vi "Reference.vi"(0 "file path (IN)":path, 1 "Project #":string, 2 "Request #":string, 3 "TEST #":string, 5 "error in (no error)":errorcluster, 6 "ICE":dbl) -> (7 "Ta (ns)":dbl, 9 "Tb (ns)":dbl, 11 "Irrm(A)":dbl, 13 "Erec (uj)":dbl, 14 "file path (OUT)":path, 15 "TRR (ns)":dbl, 16 "QRR (nc)":dbl, 17 "DONE":bool, 19 "error out":errorcluster)   [LabVIEW 2020]
uses:
  <vilib>/Analysis/NI_AALBase.lvlib
  <vilib>/measure/NI_MAPro.lvlib
  <vilib>/measure/mamon.llb/Trigger Detection for 1 Channel.vi
  <vilib>/Analysis/NI_AALPro.lvlib
  <vilib>/Analysis/1siggen.llb/Ramp Pattern by Samples.vi
panel:
  out "Erec: X-axis":dbl[](array[numeric])
  out "Erec: Y-axis":dbl[](array[numeric])
  out "Erec  : XY Graph":cluster{"X":dbl, "Y":dbl}[](graph)
  out "QRR Part2(RAMP): X-axis":dbl[](array[numeric])
  out "QRR Part2(RAMP): Y-axis":dbl[](array[numeric])
  out "QRR Part2(RAMP) : XY Graph":cluster{"X":dbl, "Y":dbl}[](graph)
  out "x-intercept of RAMP":dbl
  out "y-intercept":dbl
  out "slope":dbl
  out "QRR Part1(ICE): X-axis":dbl[](array[numeric])
  out "QRR Part1(ICE) : XY Graph":cluster{"X":dbl, "Y":dbl}[](graph)
  out "QRR Part1(ICE): Y-axis":dbl[](array[numeric])
  in  "Decision ?":bool
  out "25% Irrm Rise Edge":dbl
  out "0% Ice-Fall Edge":dbl
  out "Cursor a : Channel 1":dbl
  out "Cursor b : Channel 1":dbl
  out "Waveform Graph":waveform(dbl)[](graph)
  out "ON Region":waveform(dbl)[](graph) caption="Erec(uj)"
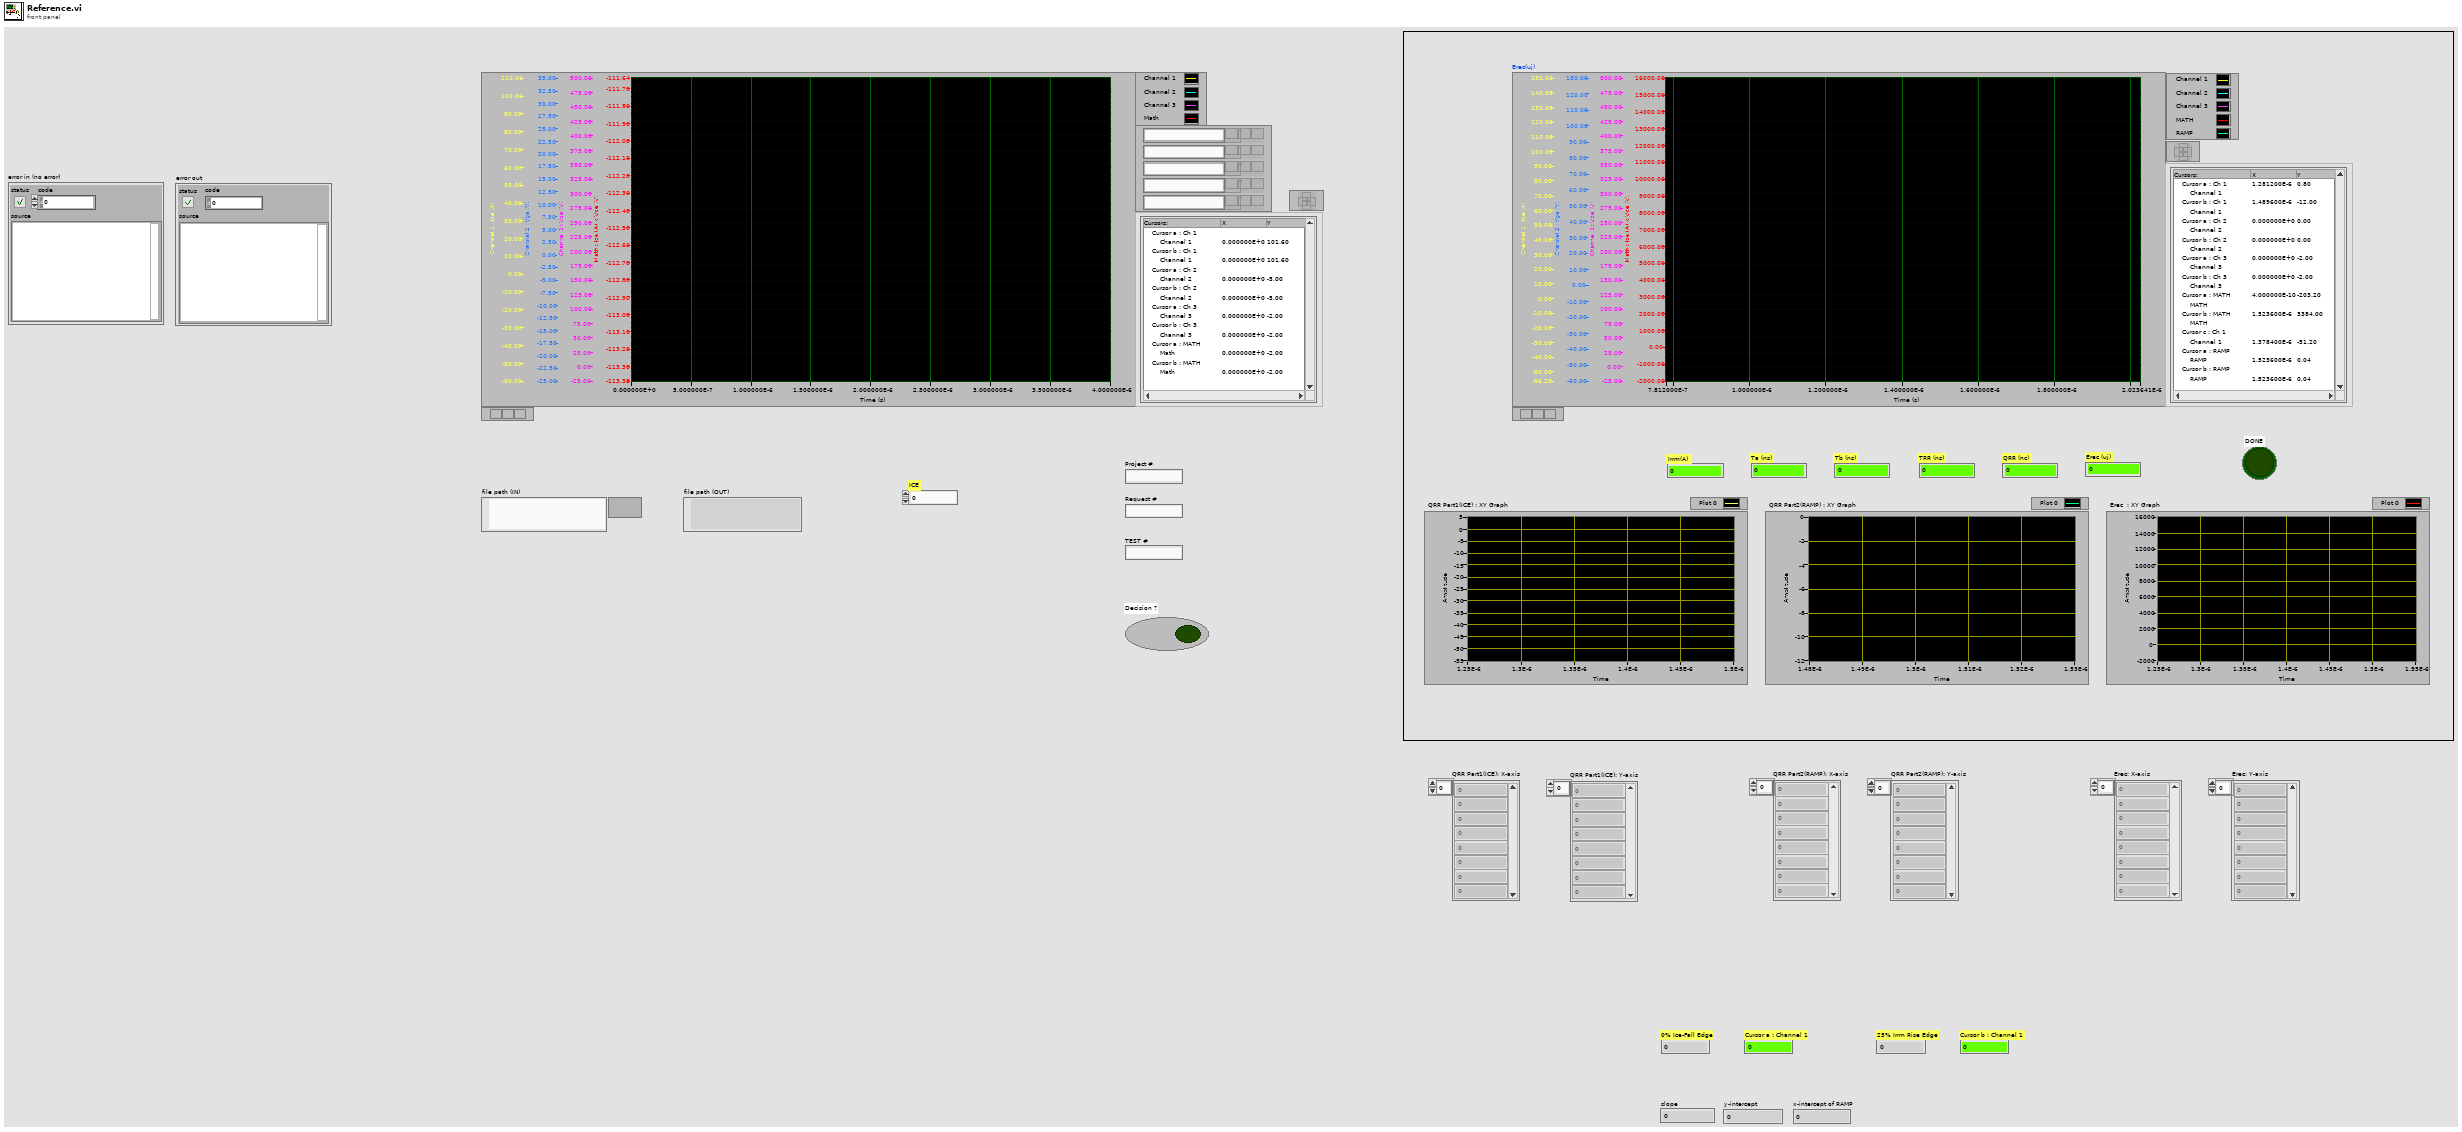
[diagram p1: front panel]
types:
  T1 = enum32{"Invalid", "Standard", "Closed", "Hidden", "Minimized", "Maximized"}
  T2 = typedef "imagedata.ctl" = cluster{"image type":i32, "image depth":i32, "image":u8[], "mask":u8[], "colors":u32[], "Rectangle":cluster{"left":i16, "top":i16, "right":i16, "bottom":i16}}
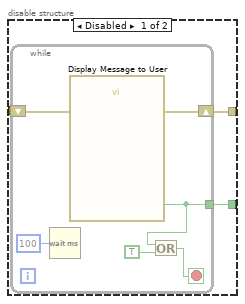
[diagram p3: hidden frame]
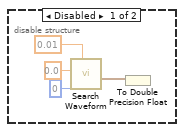
[diagram p7: hidden frame]
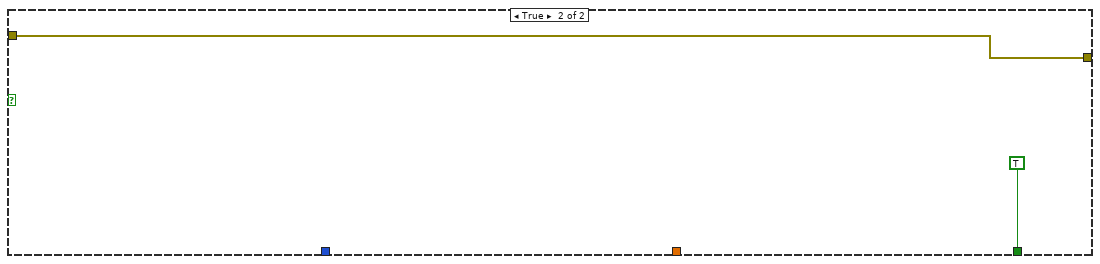
[diagram p9: hidden frame]
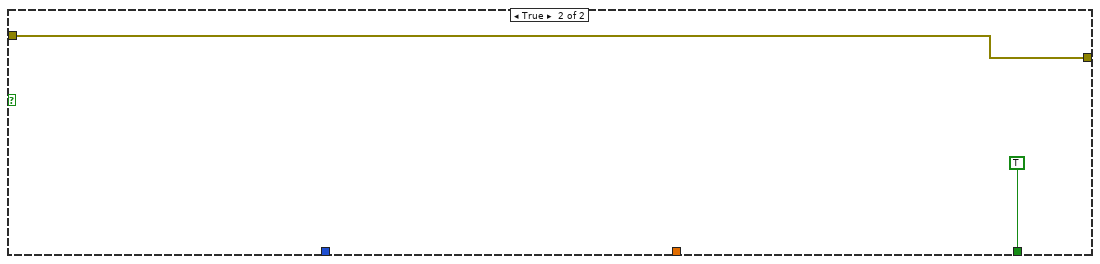
[diagram p10: hidden frame]
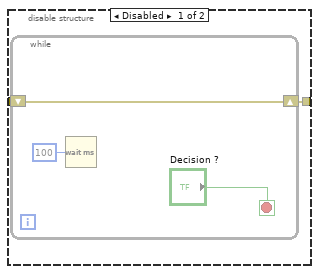
[diagram p12: hidden frame]
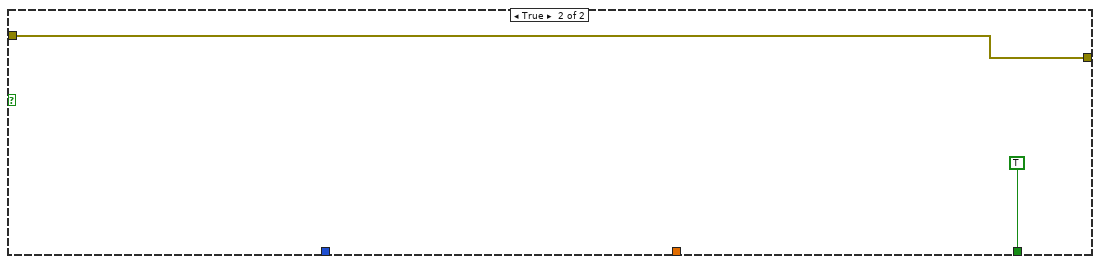
[diagram p13: hidden frame]
diagram:
  w31 = FALSE ("DONE Tdon")
  w16 = 0.0 ("Cursor a : Channel 1")
  w32 = errorcluster {"status"=FALSE, "code"=0, "source"=""} ("error out")
  w33 = waveform(dbl)[] [] ("Waveform Graph")
  n1 = local write "Cursor a : Channel 1"(w16) -> ()
  n2 = local write "Cursor b : Channel 1"(w16) -> ()
  n3 = local write "Decision ?"(w31) -> ()
  n4 = local write "error out"(w32) -> ()
  n5 = local write "error in (no error)"(w32) -> ()
  n6 = local write "DONE"(w31) -> ()
  n7 = local write "TRR (ns)"(w16) -> ()
  n8 = local write "QRR (nc)"(w16) -> ()
  n9 = local write "Waveform Graph"(w33) -> ()
  n10 = local write "ON Region"(w33) -> ()
  n11 = local write "Tb (ns)"(w16) -> ()
  n12 = local write "Erec (uj)"(w16) -> ()
  n13 = local write "Ta (ns)"(w16) -> ()
  n14 = local write "Irrm(A)"(w16) -> ()
  n15 = flat-sequence {
    tunnel: ["file path (IN)"] -> w37
    tunnel: [w38] -> w36
    tunnel: [w53] -> w35
    tunnel: [w52] -> w34
    tunnel: w37 -> [w55]
    tunnel: w36 -> [w54]
    tunnel: [w49] -> w20
    tunnel: [w48] -> w15
    tunnel: [w47] -> w14
    tunnel: [w46] -> w13
    tunnel: [w610] -> w12
    tunnel: w35 -> [w609]
    tunnel: w34 -> [w608]
    tunnel: [w608] -> w11
    tunnel: w20 -> [w607]
    tunnel: [w607] -> w9
    tunnel: w15 -> [w606]
    tunnel: [w606] -> w7
    tunnel: [w605] -> w5
    tunnel: w14 -> [w605]
    tunnel: [w604] -> w3
    tunnel: w13 -> [w604]
    tunnel: w12 -> [w624]
    tunnel: w11 -> [w634]
    tunnel: [w634] -> w10
    tunnel: w9 -> [w633]
    tunnel: [w633] -> w8
    tunnel: w7 -> [w632]
    tunnel: [w632] -> w6
    tunnel: w5 -> [w631]
    tunnel: [w631] -> w4
    tunnel: w3 -> [w630]
    tunnel: [w630] -> w2
    tunnel: [w623] -> w1
    tunnel: [w635] -> w24
    tunnel: w10 -> [w649]
    tunnel: [w649] -> w22
    tunnel: w8 -> [w640]
    tunnel: w6 -> [w636]
    tunnel: w4 -> [w637]
    tunnel: w2 -> [w639]
    tunnel: w1 -> [w641]
    tunnel: w24 -> [w764]
    tunnel: [w762] -> w23
    tunnel: w22 -> [w777]
    tunnel: [w777] -> w21
    tunnel: w23 -> [w779]
    tunnel: w21 -> [w778]
    frame #0 {
      n16 = control-ref of="This VI"() -> (w43:refnum<vi>)
      n17 = invoke class="VI" method="FP.Open"(reference=w43, error in="error in (no error)", "Activate"=TRUE ("Activate?"), "State"=T1."Maximized") -> (error out=w44:errorcluster)  [unwired: 1 in, 4 out]
      n18 = property class="VI"(reference=w43, error in=w44, "Front Panel.Closeable"=TRUE ("Front Panel Window:Closeable")) -> (error out=w38:errorcluster)  [unwired: 1 out]
    }
    frame #1 {
      n19 = while {
        tunnel: w55 -> [w128]
        shift-right: [w123] -> w53
        shift-left: w54 -> [w127]
        tunnel: [w125] -> w52
        tunnel: [w74] -> w51
        tunnel: [w73] -> w50
        tunnel: [w71] -> w48
        tunnel: [w70] -> w47
        tunnel: [w68] -> w46
        stop <- w122 stop-if-true
        n20 = flat-sequence {
          tunnel: [w158] -> w136
          tunnel: [w159] -> w135
          tunnel: w128 -> [w159]
          tunnel: w127 -> [w158]
          tunnel: w136 -> [w245]
          tunnel: w135 -> [w242]
          tunnel: [w193] -> w134
          tunnel: [w182] -> w121
          tunnel: [w179] -> w116
          tunnel: [w162] -> w93
          tunnel: [w161] -> w74
          tunnel: [w160] -> w73
          tunnel: w134 -> [w305]
          tunnel: [w305] -> w119
          tunnel: [w290] -> w118
          tunnel: w121 -> [w274]
          tunnel: [w268] -> w117
          tunnel: w116 -> [w270]
          tunnel: [w270] -> w115
          tunnel: [w269] -> w107
          tunnel: [w268] -> w106
          tunnel: [w264] -> w105
          tunnel: [w266] -> w104
          tunnel: [w267] -> w103
          tunnel: [w266] -> w96
          tunnel: w93 -> [w265]
          tunnel: [w264] -> w80
          tunnel: w119 -> [w361]
          tunnel: [w361] -> w102
          tunnel: w118 -> [w360]
          tunnel: [w360] -> w101
          tunnel: w117 -> [w359]
          tunnel: [w359] -> w100
          tunnel: [w331] -> w99
          tunnel: w115 -> [w331]
          tunnel: [w330] -> w98
          tunnel: w107 -> [w357]
          tunnel: [w357] -> w97
          tunnel: w106 -> [w339]
          tunnel: w105 -> [w338]
          tunnel: w104 -> [w337]
          tunnel: w103 -> [w336]
          tunnel: w96 -> [w329]
          tunnel: [w329] -> w95
          tunnel: w80 -> [w328]
          tunnel: [w328] -> w78
          tunnel: w102 -> [w374]
          tunnel: [w374] -> w113
          tunnel: w101 -> [w373]
          tunnel: [w373] -> w112
          tunnel: [w365] -> w111
          tunnel: w100 -> [w372]
          tunnel: [w372] -> w110
          tunnel: w99 -> [w371]
          tunnel: [w371] -> w109
          tunnel: w98 -> [w364]
          tunnel: [w364] -> w108
          tunnel: w97 -> [w369]
          tunnel: w95 -> [w363]
          tunnel: [w363] -> w94
          tunnel: [w362] -> w79
          tunnel: w78 -> [w362]
          tunnel: w113 -> [w389]
          tunnel: [w389] -> w92
          tunnel: w112 -> [w380]
          tunnel: [w380] -> w90
          tunnel: w111 -> [w387]
          tunnel: [w385] -> w88
          tunnel: w110 -> [w388]
          tunnel: [w388] -> w86
          tunnel: w109 -> [w375]
          tunnel: [w379] -> w84
          tunnel: w108 -> [w379]
          tunnel: w94 -> [w378]
          tunnel: [w378] -> w82
          tunnel: w79 -> [w377]
          tunnel: [w377] -> w77
          tunnel: [w376] -> w76
          tunnel: [w375] -> w75
          tunnel: w92 -> [w476]
          tunnel: [w476] -> w91
          tunnel: w90 -> [w475]
          tunnel: [w475] -> w89
          tunnel: w88 -> [w466]
          tunnel: [w465] -> w87
          tunnel: w86 -> [w474]
          tunnel: [w474] -> w85
          tunnel: w84 -> [w473]
          tunnel: [w473] -> w83
          tunnel: w82 -> [w472]
          tunnel: [w472] -> w81
          tunnel: w77 -> [w463]
          tunnel: w76 -> [w460]
          tunnel: w75 -> [w459]
          tunnel: [w459] -> w68
          tunnel: [w555] -> w133
          tunnel: w91 -> [w558]
          tunnel: [w558] -> w132
          tunnel: w89 -> [w557]
          tunnel: [w557] -> w131
          tunnel: w87 -> [w556]
          tunnel: w85 -> [w552]
          tunnel: [w552] -> w120
          tunnel: [w553] -> w114
          tunnel: w83 -> [w553]
          tunnel: w81 -> [w551]
          tunnel: w133 -> [w585]
          tunnel: w132 -> [w588]
          tunnel: [w588] -> w130
          tunnel: w131 -> [w575]
          tunnel: [w585] -> w129
          tunnel: w120 -> [w577]
          tunnel: w114 -> [w574]
          tunnel: [w575] -> w72
          tunnel: [w574] -> w69
          tunnel: w130 -> [w595]
          tunnel: w129 -> [w597]
          tunnel: [w596] -> w124
          tunnel: [w595] -> w125
          tunnel: w72 -> [w594]
          tunnel: [w594] -> w71
          tunnel: [w593] -> w70
          tunnel: w69 -> [w593]
          frame #0 {
            w155 = waveform(dbl)[] [] ("Waveform Graph")
            w151 = 0.0 ("Cursor a : Channel 1")
            w157 = FALSE ("DONE Tdon")
            n21 = local write "Cursor a : Channel 1"(w151) -> ()
            n22 = local write "TRR (ns)"(w151) -> ()
            n23 = local write "Cursor b : Channel 1"(w151) -> ()
            n24 = local write "Decision ?"(w157) -> ()
            n25 = local write "QRR (nc)"(w151) -> ()
            n26 = local write "Tb (ns)"(w151) -> ()
            n27 = local write "Irrm(A)"(w151) -> ()
            n28 = local write "Ta (ns)"(w151) -> ()
            n29 = local write "DONE"(w157) -> ()
            n30 = local write "QRR Part2(RAMP) : XY Graph"(cluster{"X":dbl, "Y":dbl}[] [] ("QRR : XY Graph")) -> ()
            n31 = local write "QRR Part2(RAMP): X-axis"(dbl[] [] ("QRR Area Y-axis")) -> ()
            n32 = local write "QRR Part2(RAMP): Y-axis"(dbl[] [] ("QRR Area X-axis")) -> ()
            n33 = local write "QRR Part1(ICE) : XY Graph"(cluster{"X":dbl, "Y":dbl}[] [] ("QRR : XY Graph")) -> ()
            n34 = local write "QRR Part1(ICE): Y-axis"(dbl[] [] ("QRR Area Y-axis")) -> ()
            n35 = local write "QRR Part1(ICE): X-axis"(dbl[] [] ("QRR Area X-axis")) -> ()
            n36 = Wait (ms)(milliseconds to wait=u32 200) -> ()  [unwired: 1 out]
            n37 = local write "Waveform Graph"(w155) -> ()
            n38 = local write "ON Region"(w155) -> ()
          }
          frame #1 {
            w183 = 0.0 ("number")
            w168 = waveform(dbl) {"t0"=timestamp(0 s since 1904-01-01), "dt"=1.0, "Y"=[]} ("element")
            # "t0"
            # "Channel 1"
            # "Channel 3"
            # "dt"
            # "Ch1"
            n39 = call "3_ReadDatatoWaveform.vi"("error in (no error)"=w245, "file path (IN)"=w242) -> ("error out"=w184:errorcluster, "Waveform Graph"=→"Waveform Graph":waveform(dbl)[], "file path (OUT)"=w193:path, "dt"=w179:dbl, "Ch 3 Data"=w243:dbl[], "Ch 1 Data"=w188:dbl[])  [unwired: 3 in, 1 out]
            n40 = To Time Stamp(1:w183) -> (0:w187:timestamp)
            n41 = disable-structure shown="Enabled" {
              disable-tunnel: w187 -> [w256 _]
              disable-tunnel: w179 -> [w255 _]
              disable-tunnel: w188 -> [w254 _]
              disable-tunnel: [w253 _] -> w161
              frame Enabled {
                # "Channel 1"
                n42 = Bundle By Name("Y"=w254, "dt"=w255, "t0"=w256) -> (w253:waveform(dbl))  [unwired: 1 in]
              }
              frame Disabled {
              }
            }
            n43 = disable-structure shown="Enabled" {
              disable-tunnel: w187 -> [w260 _]
              disable-tunnel: w179 -> [w259 _]
              disable-tunnel: w243 -> [w258 _]
              disable-tunnel: [w257 _] -> w160
              frame Enabled {
                # "Channel 3"
                n44 = Bundle By Name("Y"=w258, "dt"=w259, "t0"=w260) -> (w257:waveform(dbl))  [unwired: 1 in]
              }
              frame Disabled {
              }
            }
            n45 = property on="Waveform Graph" class="WFGraph (strict)"(error in=w184, "XScale.Offset"=w183) -> (error out=w181:errorcluster)  [unwired: 1 in, 1 out]
            n46 = disable-structure shown="Enabled" {
              disable-tunnel: w161 -> [w250 _]
              disable-tunnel: [w248 _] -> w189
              disable-tunnel: [w247 _] -> w182
              disable-tunnel: w181 -> [w248 _]
              disable-tunnel: w179 -> [w246 _]
              frame Enabled {
                w249 = 1 ("left rank")
                # "old = 30"
                # "Median"
                n47 = Unbundle By Name(w250) -> ("Y"=w252:dbl[])
                n48 = call <vilib>:"Median Filter.vi"("right rank"=w249, "left rank"=w249, "X"=w252) -> ("Filtered X"=w251:dbl[])  [unwired: 7 in, 1 out]
                n49 = Bundle By Name("Y"=w251, "dt"=w246) -> (w247:waveform(dbl))  [unwired: 1 in]
              }
              frame Disabled {
              }
            }
            n50 = Build Array(w161, w168, w160, w168, w168) -> (→"ON Region":waveform(dbl)[])
            n51 = Merge Errors(w181, w181, w189) -> (w200:errorcluster)
            n52 = property on="ON Region" class="WFGraph (strict)"(error in=w200) -> (error out=w199:errorcluster, "Width"=w198:u32)  [unwired: 1 in, 1 out]
            n53 = property on="ON Region" class="WFGraph (strict)"(error in=w199, "Caption.Justify"=enum16{"Left", "Center", "Right"}."Left" ("Caption.Justification"), "Caption.Width"=w198, "Caption.FontBold"=TRUE ("Caption.Font:Bold"), "Caption.FontColor"=u32 16860 ("Caption.Font:Color"), "Caption.FontSize"=u32 24 ("Caption.Font:Size"), "Caption.Text"="Irrm, Ta, Tb, TRR, QRR") -> (error out=w186:errorcluster)  [unwired: 1 in, 1 out]
            n54 = property on="ON Region" class="WFGraph (strict)"(error in=w186, "XScale.Offset"=w183) -> (error out=w185:errorcluster)  [unwired: 1 in, 1 out]
            n55 = property on="ON Region" class="WFGraph (strict)"(error in=w185, "Active Cursor"=u32 0, "Cursor.Cursor X"=0.0 ("Cursor.Cursor Position:Cursor X"), "Cursor.Cursor Y"=0.0 ("Cursor.Cursor Position:Cursor Y"), "Cursor.Visible"=FALSE) -> (error out=w224:errorcluster)  [unwired: 1 in, 1 out]
            n56 = property on="ON Region" class="WFGraph (strict)"(error in=w224, "Active Cursor"=u32 1, "Cursor.Cursor X"=0.0 ("Cursor.Cursor Position:Cursor X"), "Cursor.Cursor Y"=0.0 ("Cursor.Cursor Position:Cursor Y"), "Cursor.Visible"=FALSE) -> (error out=w223:errorcluster)  [unwired: 1 in, 1 out]
            n57 = property on="ON Region" class="WFGraph (strict)"(error in=w223, "Active Cursor"=u32 2, "Cursor.Cursor X"=0.0 ("Cursor.Cursor Position:Cursor X"), "Cursor.Cursor Y"=0.0 ("Cursor.Cursor Position:Cursor Y"), "Cursor.Visible"=FALSE) -> (error out=w222:errorcluster)  [unwired: 1 in, 1 out]
            n58 = property on="ON Region" class="WFGraph (strict)"(error in=w222, "Active Cursor"=u32 3, "Cursor.Cursor X"=0.0 ("Cursor.Cursor Position:Cursor X"), "Cursor.Cursor Y"=0.0 ("Cursor.Cursor Position:Cursor Y"), "Cursor.Visible"=FALSE) -> (error out=w205:errorcluster)  [unwired: 1 in, 1 out]
            n59 = property on="ON Region" class="WFGraph (strict)"(error in=w205, "Active Cursor"=u32 4, "Cursor.Cursor X"=0.0 ("Cursor.Cursor Position:Cursor X"), "Cursor.Cursor Y"=0.0 ("Cursor.Cursor Position:Cursor Y"), "Cursor.Visible"=FALSE) -> (error out=w204:errorcluster)  [unwired: 1 in, 1 out]
            n60 = property on="ON Region" class="WFGraph (strict)"(error in=w204, "Active Cursor"=u32 5, "Cursor.Cursor X"=0.0 ("Cursor.Cursor Position:Cursor X"), "Cursor.Cursor Y"=0.0 ("Cursor.Cursor Position:Cursor Y"), "Cursor.Visible"=FALSE) -> (error out=w203:errorcluster)  [unwired: 1 in, 1 out]
            n61 = property on="ON Region" class="WFGraph (strict)"(error in=w203, "Active Cursor"=u32 6, "Cursor.Cursor X"=0.0 ("Cursor.Cursor Position:Cursor X"), "Cursor.Cursor Y"=0.0 ("Cursor.Cursor Position:Cursor Y"), "Cursor.Visible"=FALSE) -> (error out=w202:errorcluster)  [unwired: 1 in, 1 out]
            n62 = property on="ON Region" class="WFGraph (strict)"(error in=w202, "Active Cursor"=u32 7, "Cursor.Cursor X"=0.0 ("Cursor.Cursor Position:Cursor X"), "Cursor.Cursor Y"=0.0 ("Cursor.Cursor Position:Cursor Y"), "Cursor.Visible"=FALSE) -> (error out=w170:errorcluster)  [unwired: 1 in, 1 out]
            n63 = Wait (ms)(milliseconds to wait=u32 300) -> ()  [unwired: 1 out]
            n64 = call <vilib>:"Beep.vi"("use system alert? (T)"=FALSE, "duration (msec)"=u32 200, "frequency (Hz)"=u32 2000) -> ()  [unwired: 9 in]
            n65 = property on="ON Region" class="WFGraph (strict)"(error in=w170, "Active Cursor"=u32 8, "Cursor.Cursor X"=0.0 ("Cursor.Cursor Position:Cursor X"), "Cursor.Cursor Y"=0.0 ("Cursor.Cursor Position:Cursor Y"), "Cursor.Visible"=FALSE) -> (error out=w169:errorcluster)  [unwired: 1 in, 1 out]
            n66 = property on="ON Region" class="WFGraph (strict)"(error in=w169, "Active Cursor"=u32 9, "Cursor.Cursor X"=0.0 ("Cursor.Cursor Position:Cursor X"), "Cursor.Cursor Y"=0.0 ("Cursor.Cursor Position:Cursor Y"), "Cursor.Visible"=FALSE) -> (error out=w163:errorcluster)  [unwired: 1 in, 1 out]
            n67 = property on="ON Region" class="WFGraph (strict)"(error in=w163, "Active Cursor"=u32 10, "Cursor.Cursor X"=0.0 ("Cursor.Cursor Position:Cursor X"), "Cursor.Cursor Y"=0.0 ("Cursor.Cursor Position:Cursor Y"), "Cursor.Visible"=FALSE) -> (error out=w162:errorcluster)  [unwired: 1 in, 1 out]
          }
          frame #2 {
            w287 = u16 1 items=["Falling Edge", "Rising Edge"] ("trigger slope")
            w288 = u16 1 items=["Index", "Time"] ("location mode")
            w293 = u16 0 items=["Falling Edge", "Rising Edge"] ("trigger slope")
            w294 = u16 1 items=["Index", "Time"] ("location mode")
            # "Cursor b : Channel 1"
            # "25% IRRM"
            # "Cursor c : Channel 1"
            # "Cursor c : Channel 1"
            # "Cursor a : Channel 1"
            # "Cursor b : Channel 1"
            # "Cursor a : Channel 1"
            # "Cursor b : Channel 1"
            # "Cursor a : Channel 1"
            # "Cursor b : Channel 1"
            # "Cursor a : Channel 1"
            # "End Time 1st Cursor"
            # "Point A"
            # "1st PARAMETER : 0% Ice"
            # "Channel 1"
            # "Channel 1"
            n68 = call <vilib>:"Waveform Min Max.vi"("error in (no error)"=w265, "waveform in"=w274) -> ("error out"=w279:errorcluster, "min time"=w283:timestamp)  [unwired: 4 in, 4 out]
            n69 = To Double Precision Float(number=w283) -> (double precision float=w268:dbl)
            n70 = property on="ON Region" class="WFGraph (strict)"(error in=w279, "Active Cursor"=u32 8, "Cursor.Cursor X"=w268, "Cursor.Visible"=TRUE, "Cursor.Cursor Name Visible"=TRUE) -> (error out=w277:errorcluster)  [unwired: 1 in, 1 out]
            n71 = property on="ON Region" class="WFGraph (strict)"(error in=w277, "Active Cursor"=u32 8) -> (error out=w275:errorcluster, "Cursor.Cursor Y"=w266:dbl)  [unwired: 1 in, 1 out]
            n72 = Absolute Value(x=w266) -> (abs(x)=→"Irrm(A)":dbl)
            n73 = Divide(x=0.0, y=100.0) -> (x/y=w312:dbl)
            n74 = Multiply(x=w312, y="ICE") -> (x*y=w291:dbl)
            "0% Ice-Fall Edge" <- w291
            n75 = Add(x=w291, y=0.2) -> (x+y=w261:dbl)
            n76 = call-poly <vilib>:"Basic Level Trigger Detection.vi"("signal in"=w274, "level"=w261, "hysteresis"=w261, "location mode"=w294, "error in (no error)"=w275, "trigger slope"=w293) -> ("trigger location"=w290:dbl, "error out"=w289:errorcluster)  [unwired: 7 in, 1 out]
            n77 = property on="ON Region" class="WFGraph (strict)"(error in=w289, "Active Cursor"=u32 0, "Cursor.Cursor X"=w290, "Cursor.Visible"=TRUE, "Cursor.Cursor Name Visible"=TRUE) -> (error out=w301:errorcluster)  [unwired: 1 in, 1 out]
            n78 = property on="ON Region" class="WFGraph (strict)"(error in=w301, "Active Cursor"=u32 0) -> (error out=w285:errorcluster, "Cursor.Cursor Y"=→"Cursor a : Channel 1":dbl)  [unwired: 1 in, 1 out]
            n79 = Divide(x=w266, y=4.0) -> (x/y=w273:dbl)
            "25% Irrm Rise Edge" <- w273
            n80 = Add(x=w273, y=0.2) -> (x+y=w263:dbl)
            n81 = call-poly <vilib>:"Basic Level Trigger Detection.vi"("signal in"=w274, "level"=w263, "hysteresis"=w263, "location mode"=w288, "error in (no error)"=w285, "trigger slope"=w287) -> ("trigger location"=w264:dbl, "error out"=w284:errorcluster)  [unwired: 7 in, 1 out]
            n82 = property on="ON Region" class="WFGraph (strict)"(error in=w284, "Active Cursor"=u32 1, "Cursor.Cursor X"=w264, "Cursor.Visible"=TRUE, "Cursor.Cursor Name Visible"=TRUE) -> (error out=w298:errorcluster)  [unwired: 1 in, 1 out]
            n83 = property on="ON Region" class="WFGraph (strict)"(error in=w298, "Active Cursor"=u32 1) -> (error out=w269:errorcluster, "Cursor.Cursor Y"=w267:dbl)  [unwired: 1 in, 1 out]
            "Cursor b : Channel 1" <- w267
            n84 = Wait (ms)(milliseconds to wait=u32 300) -> ()  [unwired: 1 out]
            n85 = call <vilib>:"Beep.vi"("use system alert? (T)"=FALSE, "duration (msec)"=u32 200, "frequency (Hz)"=u32 2000) -> ()  [unwired: 9 in]
            n86 = disable-structure shown="Enabled" {
              frame Disabled {
                n87 = call <vilib>:"Search Waveform.vi"("tolerance (%)"=0.01, "start index"=0, "value"=0.0) -> ("error out"=w313:errorcluster, "time of best fit"=w317:timestamp, "error in (no error)"=w314:errorcluster, "waveform in"=w318:waveform(dbl))  [unwired: 1 in, 4 out]
                n88 = To Double Precision Float(number=w317) -> ()  [unwired: 1 out]
              }
              frame Enabled {
              }
            }
            n89 = disable-structure shown="Disabled" {
              frame Disabled {
                w321 = u16 1 items=["Index", "Time"] ("location mode")
                w327 = u16 1 items=["Falling Edge", "Rising Edge"] ("trigger slope")
                # "Point B"
                n90 = call-poly <vilib>:"Basic Level Trigger Detection.vi"("level"=0.0, "hysteresis"=0.3, "location mode"=w321, "trigger slope"=w327) -> ("signal in"=w320:waveform(dbl), "trigger location"=w322:dbl, "error in (no error)"=w325:errorcluster, "error out"=w323:errorcluster)  [unwired: 7 in, 1 out]
              }
              frame Enabled {
              }
            }
          }
          frame #3 {
            w340 = 10000 ("samples")
            # "Slope"
            # "Intercept"
            # "x-axis"
            # "y-axis"
            n91 = Build Array(w339, w338) -> (w348:dbl[])
            n92 = Build Array(w337, w336) -> (w347:dbl[])
            n93 = call <vilib>:"Linear Fit.vi"("Y"=w347, "X"=w348) -> ("slope"=w356:dbl, "intercept"=w354:dbl)  [unwired: 9 in, 3 out]
            "slope" <- w356
            "y-intercept" <- w354
            n94 = Negate(x=w354) -> (-x=w355:dbl)
            n95 = Divide(x=w355, y=w356) -> (x/y=w330:dbl)
            n96 = Multiply(x=w340, y=w331) -> (x*y=w350:dbl)
            n97 = Multiply(x=w350, y=w356) -> (x*y=w351:dbl)
            n98 = Add(x=w351, y=w354) -> (x+y=w352:dbl)
            n99 = call-poly <vilib>:"Ramp Pattern.vi"("start"=w354, "end"=w352, "samples"=w340) -> ("Ramp Pattern"=w349:dbl[])  [unwired: 7 in, 1 out]
            n100 = Bundle By Name("Y"=w349, "dt"=w331) -> (w353:waveform(dbl))  [unwired: 1 in]
            n101 = local read "ON Region"() -> (w341:waveform(dbl)[])
            n102 = Index Array(array=w341, index=0) -> (element=w342:waveform(dbl))
            n103 = Index Array(array=w341, index=1) -> (element=w343:waveform(dbl))
            n104 = Index Array(array=w341, index=2) -> (element=w344:waveform(dbl))
            n105 = Index Array(array=w341, index=3) -> (element=w345:waveform(dbl))
            n106 = Build Array(w342, w343, w344, w345, w353) -> (w346:waveform(dbl)[])
            n107 = local write "ON Region"(w346) -> ()
            n108 = Wait (ms)(milliseconds to wait=u32 400) -> ()  [unwired: 1 out]
          }
          frame #4 {
            # "x-intercept of RAMP"
            # "Cursor a : Channel RAMP"
            n109 = property on="ON Region" class="WFGraph (strict)"(error in=w369, "Active Cursor"=u32 9, "Cursor.Cursor X"=w364, "Cursor.Visible"=TRUE, "Cursor.Cursor Name Visible"=TRUE) -> (error out=w365:errorcluster)  [unwired: 1 in, 1 out]
            n110 = Wait (ms)(milliseconds to wait=u32 400) -> ()  [unwired: 1 out]
            "x-intercept of RAMP" <- w364
          }
          frame #5 {
            # "dt"
            n111 = flat-sequence {
              tunnel: w387 -> [w392]
              tunnel: w375 -> [w391]
              tunnel: [w390] -> w386
              tunnel: w386 -> [w435]
              tunnel: [w435] -> w384
              tunnel: [w434] -> w383
              tunnel: [w433] -> w382
              tunnel: w384 -> [w443]
              tunnel: w383 -> [w442]
              tunnel: w382 -> [w441]
              tunnel: [w443] -> w381
              tunnel: [w438] -> w376
              tunnel: [w456] -> w385
              tunnel: w381 -> [w457]
              tunnel: w380 -> [w454]
              frame #0 {
                n112 = while {
                  tunnel: w392 -> [w404]
                  tunnel: w391 -> [w396]
                  tunnel: [w393] -> w390
                  i -> [w397]
                  stop <- w395 stop-if-true
                  # "Cursor b : Channel 1"
                  # "Cursor a : Channel 1"
                  n113 = property on="ON Region" class="WFGraph (strict)"(error in=w404, "Active Cursor"=u32 1) -> (error out=w402:errorcluster, "Cursor.Cursor X"=w400:dbl)  [unwired: 1 in, 1 out]
                  n114 = property on="ON Region" class="WFGraph (strict)"(error in=w404, "Active Cursor"=u32 0) -> (error out=w403:errorcluster, "Cursor.Cursor X"=w401:dbl)  [unwired: 1 in, 1 out]
                  n115 = Merge Errors(w403, w402) -> (w394:errorcluster)
                  n116 = Equal?(x=w401, y=w400) -> (x = y?=w399:bool)
                  n117 = case shown="False" w399 {
                    tunnel: w397 -> [w412 _]
                    tunnel: w396 -> [w410 _]
                    tunnel: [FALSE TRUE] -> w395
                    tunnel: w394 -> [w408 w431]
                    tunnel: [w407 w431] -> w393
                    frame False {
                      n118 = flat-sequence {
                        tunnel: w412 -> [w417]
                        tunnel: [w414] -> w411
                        tunnel: w408 -> [w413]
                        tunnel: w411 -> [w429]
                        tunnel: w410 -> [w424]
                        tunnel: [w423] -> w407
                        frame #0 {
                          # "Cursor a : Channel 1"
                          n119 = property on="ON Region" class="WFGraph (strict)"(error in=w413, "Active Cursor"=u32 0) -> (error out=w414:errorcluster, "Cursor.Cursor X"=w421:dbl, "Cursor.Cursor Y"=w420:dbl)  [unwired: 1 in, 1 out]
                          n120 = local read "QRR Part1(ICE): Y-axis"() -> (w419:dbl[])
                          n121 = local read "QRR Part1(ICE): X-axis"() -> (w418:dbl[])
                          n122 = Insert Into Array(array=w419, index=w417, new element=w420) -> (w415:dbl[])
                          n123 = Insert Into Array(array=w418, index=w417, new element=w421) -> (w416:dbl[])
                          n124 = local write "QRR Part1(ICE): X-axis"(w416) -> ()
                          n125 = local write "QRR Part1(ICE): Y-axis"(w415) -> ()
                        }
                        frame #1 {
                          # "Cursor a : Channel 1"
                          # "Cursor a : Channel 1"
                          n126 = property on="ON Region" class="WFGraph (strict)"(error in=w429, "Active Cursor"=u32 0) -> (error out=w425:errorcluster, "Cursor.Cursor X"=w428:dbl)  [unwired: 1 in, 1 out]
                          n127 = Add(x=w428, y=w424) -> (x+y=w426:dbl)
                          n128 = property on="ON Region" class="WFGraph (strict)"(error in=w425, "Active Cursor"=u32 0, "Cursor.Cursor X"=w426) -> (error out=w423:errorcluster)  [unwired: 1 in, 1 out]
                        }
                      }
                    }
                    frame True {
                    }
                  }
                  n129 = Wait (ms)(milliseconds to wait=u32 1) -> ()  [unwired: 1 out]
                }
              }
              frame #1 {
                n130 = local read "QRR Part1(ICE): X-axis"() -> (w434:dbl[])
                n131 = local read "QRR Part1(ICE): Y-axis"() -> (w433:dbl[])
                n132 = Build Cluster Array(w434, w433) -> (w437:cluster{dbl, dbl}[])
                n133 = local write "QRR Part1(ICE) : XY Graph"(w437) -> ()
                n134 = Wait (ms)(milliseconds to wait=u32 50) -> ()  [unwired: 1 out]
              }
              frame #2 {
                # "ns"
                n135 = Delete From Array(array=w442, index=0) -> (array with subset deleted=w453:dbl[])  [unwired: 1 in, 1 out]
                n136 = Delete From Array(array=w441, index=0) -> (array with subset deleted=w447:dbl[])  [unwired: 1 in, 1 out]
                n137 = Subtract(x=w453, y=w442) -> (x-y=w452:dbl[])
                n138 = Add(x=w447, y=w441) -> (x+y=w451:dbl[])
                n139 = Wait (ms)(milliseconds to wait=u32 50) -> ()  [unwired: 1 out]
                n140 = Compound Arithmetic op=MULTIPLY(w452, w451, invert 2.0 ("Numeric")) -> (w449:dbl[])
                n141 = Add Array Elements(numeric array=w449) -> (sum=w445:dbl)
                n142 = Multiply(x=w445, y=1000000000.0) -> (x*y=w439:dbl)
                n143 = Absolute Value(x=w439) -> (abs(x)=w438:dbl)
              }
              frame #3 {
                # "Cursor a : Channel 1"
                n144 = property on="ON Region" class="WFGraph (strict)"(error in=w457, "Active Cursor"=u32 0, "Cursor.Cursor X"=w454) -> (error out=w456:errorcluster)  [unwired: 1 in, 1 out]
                n145 = Wait (ms)(milliseconds to wait=u32 50) -> ()  [unwired: 1 out]
              }
            }
          }
          frame #6 {
            n146 = flat-sequence {
              tunnel: w466 -> [w479]
              tunnel: [w478] -> w464
              tunnel: w463 -> [w480]
              tunnel: w459 -> [w483]
              tunnel: [w482] -> w471
              tunnel: w464 -> [w484]
              tunnel: w471 -> [w527]
              tunnel: [w527] -> w470
              tunnel: [w526] -> w469
              tunnel: [w525] -> w468
              tunnel: w470 -> [w535]
              tunnel: w469 -> [w534]
              tunnel: w468 -> [w533]
              tunnel: [w535] -> w467
              tunnel: [w530] -> w462
              tunnel: [w548] -> w465
              tunnel: w467 -> [w549]
              frame #0 {
                # "Cursor b : RAMP"
                n147 = property on="ON Region" class="WFGraph (strict)"(error in=w479, "Active Cursor"=u32 10, "Cursor.Cursor X"=w480, "Cursor.Visible"=TRUE) -> (error out=w478:errorcluster)  [unwired: 1 in, 1 out]
              }
              frame #1 {
                n148 = while {
                  tunnel: w484 -> [w496]
                  tunnel: w483 -> [w488]
                  tunnel: [w485] -> w482
                  i -> [w489]
                  stop <- w487 stop-if-true
                  # "Cursor a : RAMP"
                  # "Cursor b : RAMP"
                  n149 = property on="ON Region" class="WFGraph (strict)"(error in=w496, "Active Cursor"=u32 9) -> (error out=w494:errorcluster, "Cursor.Cursor X"=w492:dbl)  [unwired: 1 in, 1 out]
                  n150 = property on="ON Region" class="WFGraph (strict)"(error in=w496, "Active Cursor"=u32 10) -> (error out=w495:errorcluster, "Cursor.Cursor X"=w493:dbl)  [unwired: 1 in, 1 out]
                  n151 = Merge Errors(w495, w494) -> (w486:errorcluster)
                  n152 = Equal?(x=w493, y=w492) -> (x = y?=w491:bool)
                  n153 = case shown="False" w491 {
                    tunnel: w489 -> [w504 _]
                    tunnel: w488 -> [w502 _]
                    tunnel: [FALSE TRUE] -> w487
                    tunnel: w486 -> [w500 w523]
                    tunnel: [w499 w523] -> w485
                    frame False {
                      n154 = flat-sequence {
                        tunnel: w504 -> [w509]
                        tunnel: [w506] -> w503
                        tunnel: w500 -> [w505]
                        tunnel: w503 -> [w521]
                        tunnel: w502 -> [w516]
                        tunnel: [w515] -> w499
                        frame #0 {
                          # "Cursor b : RAMP"
                          n155 = property on="ON Region" class="WFGraph (strict)"(error in=w505, "Active Cursor"=u32 10) -> (error out=w506:errorcluster, "Cursor.Cursor X"=w513:dbl, "Cursor.Cursor Y"=w512:dbl)  [unwired: 1 in, 1 out]
                          n156 = local read "QRR Part2(RAMP): Y-axis"() -> (w511:dbl[])
                          n157 = local read "QRR Part2(RAMP): X-axis"() -> (w510:dbl[])
                          n158 = Insert Into Array(array=w511, index=w509, new element=w512) -> (w507:dbl[])
                          n159 = Insert Into Array(array=w510, index=w509, new element=w513) -> (w508:dbl[])
                          n160 = local write "QRR Part2(RAMP): X-axis"(w508) -> ()
                          n161 = local write "QRR Part2(RAMP): Y-axis"(w507) -> ()
                        }
                        frame #1 {
                          # "Cursor b : RAMP"
                          # "Cursor b : RAMP"
                          n162 = property on="ON Region" class="WFGraph (strict)"(error in=w521, "Active Cursor"=u32 10) -> (error out=w517:errorcluster, "Cursor.Cursor X"=w520:dbl)  [unwired: 1 in, 1 out]
                          n163 = Add(x=w520, y=w516) -> (x+y=w518:dbl)
                          n164 = property on="ON Region" class="WFGraph (strict)"(error in=w517, "Active Cursor"=u32 10, "Cursor.Cursor X"=w518) -> (error out=w515:errorcluster)  [unwired: 1 in, 1 out]
                        }
                      }
                    }
                    frame True {
                    }
                  }
                  n165 = Wait (ms)(milliseconds to wait=u32 1) -> ()  [unwired: 1 out]
                }
              }
              frame #2 {
                n166 = local read "QRR Part2(RAMP): X-axis"() -> (w526:dbl[])
                n167 = local read "QRR Part2(RAMP): Y-axis"() -> (w525:dbl[])
                n168 = Build Cluster Array(w526, w525) -> (w529:cluster{dbl, dbl}[])
                n169 = Wait (ms)(milliseconds to wait=u32 50) -> ()  [unwired: 1 out]
                n170 = local write "QRR Part2(RAMP) : XY Graph"(w529) -> ()
              }
              frame #3 {
                # "ns"
                n171 = Delete From Array(array=w534, index=0) -> (array with subset deleted=w545:dbl[])  [unwired: 1 in, 1 out]
                n172 = Delete From Array(array=w533, index=0) -> (array with subset deleted=w539:dbl[])  [unwired: 1 in, 1 out]
                n173 = Subtract(x=w545, y=w534) -> (x-y=w544:dbl[])
                n174 = Add(x=w539, y=w533) -> (x+y=w543:dbl[])
                n175 = Wait (ms)(milliseconds to wait=u32 50) -> ()  [unwired: 1 out]
                n176 = Compound Arithmetic op=MULTIPLY(w544, w543, invert 2.0 ("Numeric")) -> (w541:dbl[])
                n177 = Add Array Elements(numeric array=w541) -> (sum=w537:dbl)
                n178 = Multiply(x=w537, y=1000000000.0) -> (x*y=w531:dbl)
                n179 = Absolute Value(x=w531) -> (abs(x)=w530:dbl)
              }
              frame #4 {
                # "Cursor b : RAMP"
                n180 = property on="ON Region" class="WFGraph (strict)"(error in=w549, "Active Cursor"=u32 10, "Cursor.Visible"=FALSE) -> (error out=w548:errorcluster)  [unwired: 1 in, 1 out]
                n181 = Wait (ms)(milliseconds to wait=u32 50) -> ()  [unwired: 1 out]
              }
            }
            n182 = Add(x=w460, y=w462) -> (x+y=→"QRR (nc)":dbl)
          }
          frame #7 {
            n183 = disable-structure shown="Enabled" {
              disable-tunnel: w556 -> [w573 _]
              disable-tunnel: [w572 _] -> w555
              disable-tunnel: w557 -> [w567 _]
              disable-tunnel: w553 -> [w566 _]
              disable-tunnel: w551 -> [w560 _]
              frame Enabled {
                # "2nd Cursor"
                # "1st Cursor"
                n184 = local read "ICE"() -> (w564:dbl)
                n185 = Subtract(x=w567, y=5e-07) -> (x-y=w568:dbl)
                n186 = Subtract(x=w560, y=5.0) -> (x-y=w559:dbl)
                n187 = Add(x=w566, y=5e-07) -> (x+y=w569:dbl)
                n188 = Divide(x=w564, y=2.0) -> (x/y=w562:dbl)
                n189 = property on="ON Region" class="WFGraph (strict)"(error in=w573, "XScale.Minimum"=w568, "XScale.Maximum"=w569, "ActYScl"=0 ("Active Y Scale"), "YScale.Minimum"=w559, "YScale.Maximum"=w562) -> (error out=w572:errorcluster)  [unwired: 1 in, 1 out]
              }
              frame Disabled {
              }
            }
            n190 = Wait (ms)(milliseconds to wait=u32 300) -> ()  [unwired: 1 out]
          }
          frame #8 {
            # "ns"
            # "Cursor a : RAMP"
            # "Cursor a : Channel 1"
            # "Cursor c : Channel 1"
            # "ns"
            n191 = Subtract(x=w577, y=w575) -> (x-y=w587:dbl)
            n192 = Subtract(x=w574, y=w577) -> (x-y=w583:dbl)
            n193 = Absolute Value(x=w587) -> (abs(x)=w586:dbl)
            n194 = Absolute Value(x=w583) -> (abs(x)=w584:dbl)
            n195 = Multiply(x=w586, y=1000000000.0) -> (x*y=w580:dbl)
            "Ta (ns)" <- w580
            n196 = Multiply(x=w584, y=1000000000.0) -> (x*y=w579:dbl)
            "Tb (ns)" <- w579
            n197 = Add(x=w580, y=w579) -> (x+y=w581:dbl)
            n198 = Wait (ms)(milliseconds to wait=u32 300) -> ()  [unwired: 1 out]
            n199 = call <vilib>:"Beep.vi"("use system alert? (T)"=FALSE, "duration (msec)"=u32 200, "frequency (Hz)"=u32 2000) -> ()  [unwired: 9 in]
            n200 = Absolute Value(x=w581) -> (abs(x)=→"TRR (ns)":dbl)
          }
          frame #9 {
            n201 = disable-structure shown="Enabled" {
              disable-tunnel: w597 -> [w599 w603]
              disable-tunnel: [w598 w603] -> w596
              frame Disabled {
                n202 = while {
                  shift-right: [w600] -> w598
                  shift-left: w599 -> [w600]
                  stop <- "Decision ?" stop-if-true
                  n203 = Wait (ms)(milliseconds to wait=u32 100) -> ()  [unwired: 1 out]
                }
              }
              frame Enabled {
              }
            }
          }
        }
        n204 = disable-structure shown="Enabled" {
          disable-tunnel: w124 -> [w139 w146]
          disable-tunnel: [w138 w146] -> w123
          disable-tunnel: [w137 TRUE ("NO")] -> w122
          frame Disabled {
            n205 = while {
              tunnel: [w141] -> w137
              shift-right: [w144] -> w138
              shift-left: w139 -> [w145]
              stop <- w143 stop-if-true
              n206 = Wait (ms)(milliseconds to wait=u32 100) -> ()  [unwired: 1 out]
              n207 = call "Display Message to User"("error in (no error)"=w145) -> ("error out"=w144:errorcluster, "NO"=w141:bool)  [unwired: 9 in]
              n208 = Or(x=w141, y=TRUE) -> (x .or. y?=w143:bool)
            }
          }
          frame Enabled {
          }
        }
        n209 = Wait (ms)(milliseconds to wait=u32 100) -> ()  [unwired: 1 out]
      }
      n210 = disable-structure shown="Enabled" {
        disable-tunnel: w51 -> [w58 _]
        disable-tunnel: w50 -> [w57 _]
        disable-tunnel: [w56 _] -> w49
        frame Enabled {
          # "Channel 3"
          # "Channel 1"
          # "MATH = - Ch1 x Ch3"
          n211 = Unbundle By Name(w57) -> ("Y"=w61:dbl[])
          n212 = Unbundle By Name(w58) -> ("Y"=w62:dbl[], "dt"=w59:dbl, "t0"=w63:timestamp)
          n213 = for {
            tunnel: w62 -> [w65] mode=indexing
            tunnel: w61 -> [w67] mode=indexing
            tunnel: [w66] -> w60 mode=indexing
            n214 = Negate(x=w65) -> (-x=w64:dbl)
            n215 = Multiply(x=w64, y=w67) -> (x*y=w66:dbl)
          }
          n216 = Bundle By Name("Y"=w60, "dt"=w59, "t0"=w63) -> (w56:waveform(dbl))  [unwired: 1 in]
        }
        frame Disabled {
        }
      }
    }
    frame #2 {
      w613 = "_"
      n217 = invoke on="ON Region" class="WFGraph (strict)" method="Get Image"(error in=w609) -> (error out=w615:errorcluster, "image data"=w618:T2)  [unwired: 5 in, 4 out]
      n218 = Concatenate Strings("C:\\TRR_Project\\TRR_Image\\" ("string"), "Project #", w613, "Request #", w613, "TEST #", w613, "TRR_QRR" ("string"), ".png" ("string")) -> (w619:string)
      n219 = String To Path(string=w619) -> (path=w617:path)
      n220 = call <vilib>:"Write PNG File.vi"("error in (no error)"=w615, "image data"=w618, "path to PNG file"=w617) -> ("error out"=w610:errorcluster)  [unwired: 7 in, 1 out]
    }
    frame #3 {
      n221 = property on="ON Region" class="WFGraph (strict)"(error in=w624, "Caption.Justify"=enum16{"Left", "Center", "Right"}."Left" ("Caption.Justification"), "Caption.FontBold"=TRUE ("Caption.Font:Bold"), "Caption.FontColor"=u32 16860 ("Caption.Font:Color"), "Caption.FontSize"=u32 24 ("Caption.Font:Size"), "Caption.Text"="Erec(uj)") -> (error out=w623:errorcluster)  [unwired: 1 in, 1 out]
      n222 = Wait (ms)(milliseconds to wait=u32 500) -> ()  [unwired: 1 out]
    }
    frame #4 {
      # "Cursor a : RAMP"
      # "Cursor a : Ch 1"
      n223 = flat-sequence {
        tunnel: w641 -> [w662]
        tunnel: [w662] -> w642
        tunnel: w640 -> [w655]
        tunnel: [w671] -> w648
        tunnel: w642 -> [w669]
        tunnel: w636 -> [w667]
        tunnel: w637 -> [w666]
        tunnel: w639 -> [w674]
        tunnel: [w673] -> w647
        tunnel: w648 -> [w675]
        tunnel: w647 -> [w718]
        tunnel: [w718] -> w646
        tunnel: [w717] -> w645
        tunnel: [w716] -> w644
        tunnel: w646 -> [w726]
        tunnel: w645 -> [w725]
        tunnel: w644 -> [w724]
        tunnel: [w726] -> w643
        tunnel: w643 -> [w740]
        tunnel: w639 -> [w737]
        tunnel: [w739] -> w638
        tunnel: w638 -> [w744]
        tunnel: w637 -> [w742]
        tunnel: w636 -> [w743]
        tunnel: [w745] -> w635
        frame #0 {
          n224 = local read "ON Region"() -> (w657:waveform(dbl)[])
          n225 = Index Array(array=w657, index=0) -> (element=w658:waveform(dbl))
          n226 = Index Array(array=w657, index=1) -> (element=w659:waveform(dbl))
          n227 = Index Array(array=w657, index=2) -> (element=w660:waveform(dbl))
          n228 = Index Array(array=w657, index=4) -> (element=w656:waveform(dbl))
          n229 = Build Array(w658, w659, w660, w655, w656) -> (w661:waveform(dbl)[])
          n230 = local write "ON Region"(w661) -> ()
          n231 = Wait (ms)(milliseconds to wait=u32 300) -> ()  [unwired: 1 out]
        }
        frame #1 {
          # "Cursor a : MATH"
          # "Cursor b : MATH"
          n232 = property on="ON Region" class="WFGraph (strict)"(error in=w669, "Active Cursor"=u32 6, "Cursor.Cursor X"=w667, "Cursor.Visible"=TRUE) -> (error out=w668:errorcluster)  [unwired: 1 in, 1 out]
          n233 = property on="ON Region" class="WFGraph (strict)"(error in=w668, "Active Cursor"=u32 7, "Cursor.Cursor X"=w666, "Cursor.Visible"=TRUE) -> (error out=w671:errorcluster)  [unwired: 1 in, 1 out]
          n234 = Wait (ms)(milliseconds to wait=u32 300) -> ()  [unwired: 1 out]
        }
        frame #2 {
          n235 = while {
            tunnel: w675 -> [w687]
            tunnel: w674 -> [w679]
            tunnel: [w676] -> w673
            i -> [w680]
            stop <- w678 stop-if-true
            # "Cursor b : MATH"
            # "Cursor a : MATH"
            n236 = property on="ON Region" class="WFGraph (strict)"(error in=w687, "Active Cursor"=u32 7) -> (error out=w685:errorcluster, "Cursor.Cursor X"=w683:dbl)  [unwired: 1 in, 1 out]
            n237 = property on="ON Region" class="WFGraph (strict)"(error in=w687, "Active Cursor"=u32 6) -> (error out=w686:errorcluster, "Cursor.Cursor X"=w684:dbl)  [unwired: 1 in, 1 out]
            n238 = Merge Errors(w686, w685) -> (w677:errorcluster)
            n239 = Equal?(x=w684, y=w683) -> (x = y?=w682:bool)
            n240 = case shown="False" w682 {
              tunnel: w680 -> [w695 _]
              tunnel: w679 -> [w693 _]
              tunnel: [FALSE TRUE] -> w678
              tunnel: w677 -> [w691 w714]
              tunnel: [w690 w714] -> w676
              frame False {
                n241 = flat-sequence {
                  tunnel: w695 -> [w700]
                  tunnel: [w697] -> w694
                  tunnel: w691 -> [w696]
                  tunnel: w694 -> [w712]
                  tunnel: w693 -> [w707]
                  tunnel: [w706] -> w690
                  frame #0 {
                    # "Cursor a : MATH"
                    n242 = property on="ON Region" class="WFGraph (strict)"(error in=w696, "Active Cursor"=u32 6) -> (error out=w697:errorcluster, "Cursor.Cursor X"=w704:dbl, "Cursor.Cursor Y"=w703:dbl)  [unwired: 1 in, 1 out]
                    n243 = local read "Erec: Y-axis"() -> (w702:dbl[])
                    n244 = local read "Erec: X-axis"() -> (w701:dbl[])
                    n245 = Insert Into Array(array=w702, index=w700, new element=w703) -> (w698:dbl[])
                    n246 = Insert Into Array(array=w701, index=w700, new element=w704) -> (w699:dbl[])
                    n247 = local write "Erec: X-axis"(w699) -> ()
                    n248 = local write "Erec: Y-axis"(w698) -> ()
                  }
                  frame #1 {
                    # "Cursor a : MATH"
                    # "Cursor a : MATH"
                    n249 = property on="ON Region" class="WFGraph (strict)"(error in=w712, "Active Cursor"=u32 6) -> (error out=w708:errorcluster, "Cursor.Cursor X"=w711:dbl)  [unwired: 1 in, 1 out]
                    n250 = Add(x=w711, y=w707) -> (x+y=w709:dbl)
                    n251 = property on="ON Region" class="WFGraph (strict)"(error in=w708, "Active Cursor"=u32 6, "Cursor.Cursor X"=w709) -> (error out=w706:errorcluster)  [unwired: 1 in, 1 out]
                  }
                }
              }
              frame True {
              }
            }
            n252 = Wait (ms)(milliseconds to wait=u32 1) -> ()  [unwired: 1 out]
          }
        }
        frame #3 {
          n253 = local read "Erec: X-axis"() -> (w717:dbl[])
          n254 = local read "Erec: Y-axis"() -> (w716:dbl[])
          n255 = Build Cluster Array(w717, w716) -> (w720:cluster{dbl, dbl}[])
          n256 = Wait (ms)(milliseconds to wait=u32 50) -> ()  [unwired: 1 out]
          n257 = local write "Erec  : XY Graph"(w720) -> ()
        }
        frame #4 {
          # "uj"
          n258 = Delete From Array(array=w725, index=0) -> (array with subset deleted=w736:dbl[])  [unwired: 1 in, 1 out]
          n259 = Delete From Array(array=w724, index=0) -> (array with subset deleted=w730:dbl[])  [unwired: 1 in, 1 out]
          n260 = Subtract(x=w736, y=w725) -> (x-y=w735:dbl[])
          n261 = Add(x=w730, y=w724) -> (x+y=w734:dbl[])
          n262 = Wait (ms)(milliseconds to wait=u32 50) -> ()  [unwired: 1 out]
          n263 = Compound Arithmetic op=MULTIPLY(w735, w734, invert 2.0 ("Numeric")) -> (w732:dbl[])
          n264 = Add Array Elements(numeric array=w732) -> (sum=w728:dbl)
          n265 = Multiply(x=w728, y=1000000.0) -> (x*y=w722:dbl)
          n266 = Absolute Value(x=w722) -> (abs(x)=→"Erec (uj)":dbl)
        }
        frame #5 {
          # "Cursor a : MATH"
          n267 = property on="ON Region" class="WFGraph (strict)"(error in=w740, "Active Cursor"=u32 6, "Cursor.Cursor X"=w737) -> (error out=w739:errorcluster)  [unwired: 1 in, 1 out]
          n268 = Wait (ms)(milliseconds to wait=u32 50) -> ()  [unwired: 1 out]
        }
        frame #6 {
          n269 = disable-structure shown="Enabled" {
            disable-tunnel: w744 -> [w761 _]
            disable-tunnel: [w760 _] -> w745
            disable-tunnel: w743 -> [w755 _]
            disable-tunnel: w742 -> [w754 _]
            frame Enabled {
              # "2nd Cursor"
              # "1st Cursor"
              n270 = local read "Irrm(A)"() -> (w746:dbl)
              n271 = Negate(x=w746) -> (-x=w747:dbl)
              n272 = local read "ICE"() -> (w752:dbl)
              n273 = Subtract(x=w755, y=5e-07) -> (x-y=w756:dbl)
              n274 = Subtract(x=w747, y=5.0) -> (x-y=w748:dbl)
              n275 = Add(x=w754, y=5e-07) -> (x+y=w757:dbl)
              n276 = Divide(x=w752, y=2.0) -> (x/y=w750:dbl)
              n277 = property on="ON Region" class="WFGraph (strict)"(error in=w761, "XScale.Minimum"=w756, "XScale.Maximum"=w757, "ActYScl"=0 ("Active Y Scale"), "YScale.Minimum"=w748, "YScale.Maximum"=w750) -> (error out=w760:errorcluster)  [unwired: 1 in, 1 out]
            }
            frame Disabled {
            }
          }
        }
      }
    }
    frame #5 {
      w767 = "_"
      n278 = Wait (ms)(milliseconds to wait=u32 300) -> ()  [unwired: 1 out]
      n279 = local read "Request #"() -> (w769:string)
      n280 = local read "Project #"() -> (w770:string)
      n281 = local read "TEST #"() -> (w771:string)
      n282 = invoke on="ON Region" class="WFGraph (strict)" method="Get Image"(error in=w764) -> (error out=w775:errorcluster, "image data"=w773:T2)  [unwired: 5 in, 4 out]
      n283 = Concatenate Strings("C:\\TRR_Project\\TRR_Image\\" ("string"), w771, w767, w770, w767, w769, w767, "Erec" ("string"), ".png" ("string")) -> (w772:string)
      n284 = String To Path(string=w772) -> (path=w774:path)
      n285 = call <vilib>:"Write PNG File.vi"("error in (no error)"=w775, "image data"=w773, "path to PNG file"=w774) -> ("error out"=w762:errorcluster)  [unwired: 7 in, 1 out]
      "DONE" <- TRUE ("DONE Tdon")
    }
    frame #6 {
      n286 = disable-structure shown="Enabled" {
        disable-tunnel: w779 -> [w780 _]
        frame Enabled {
          n287 = control-ref of="This VI"() -> (w781:refnum<vi>)
          n288 = invoke class="VI" method="FP.Close"(reference=w781, error in=w780) -> ()  [unwired: 1 in, 3 out]
        }
        frame Disabled {
        }
      }
      "error out" <- w779
      "file path (OUT)" <- w778
    }
  }
  "QRR Part1(ICE): X-axis" <- dbl[] [] ("QRR Area X-axis")
  "QRR Part1(ICE): Y-axis" <- dbl[] [] ("QRR Area Y-axis")
  "QRR Part1(ICE) : XY Graph" <- cluster{"X":dbl, "Y":dbl}[] [] ("QRR : XY Graph")
  "QRR Part2(RAMP) : XY Graph" <- cluster{"X":dbl, "Y":dbl}[] [] ("QRR Part2(RAMP) : XY Graph")
  "QRR Part2(RAMP): Y-axis" <- dbl[] [] ("QRR Part2(RAMP): Y-axis")
  "QRR Part2(RAMP): X-axis" <- dbl[] [] ("QRR Part2(RAMP): X-axis")
  "Erec  : XY Graph" <- cluster{"X":dbl, "Y":dbl}[] [] ("QRR Part2(RAMP) : XY Graph")
  "Erec: Y-axis" <- dbl[] [] ("QRR Part2(RAMP): X-axis")
  "Erec: X-axis" <- dbl[] [] ("QRR Part2(RAMP): Y-axis")
